vi "test BC to RT with Start Stop and Status.vi"(8 "error in":errorcluster, 11 "Loopback in":refnum<class "Loopback.lvclass">) -> (0 "error out":errorcluster, 3 "Loopback out":refnum<class "Loopback.lvclass">)   [LabVIEW 2020, in "Loopback.lvclass"]
uses:
  Loopback.lvclass
  C:/Users/nitest/Desktop/Git 2020/niveristand-custom-device-testing-tools/VeriStandTestCase/VeriStandTestCase.lvclass
  <vilib>/numeric/Random Number (Range) U64.vi
  8be00f4c-25bf-4da0-90d8-0b538b3cd633.vi
  2563bb73-47aa-45b7-be38-1c5e71b75716.vi
  <vilib>/numeric/sub_Random U32.vi
  <vilib>/NI VeriStand/Execution/Workspace/NI VeriStand - Set Single Channel Value.vi
  <vilib>/NI VeriStand/Execution/Workspace/NI VeriStand - Set Multiple Channel Values.vi
  <vilib>/NI VeriStand/Execution/Workspace/NI VeriStand - Get Multiple Channel Values.vi
  niveristand-custom-device-testing-tools/VeriStandTestUtilities/VeriStandTestUtilities.lvlib
  <vilib>/NI VeriStand/Execution/Workspace/NI_VS Workspace ExecutionAPI.lvlib
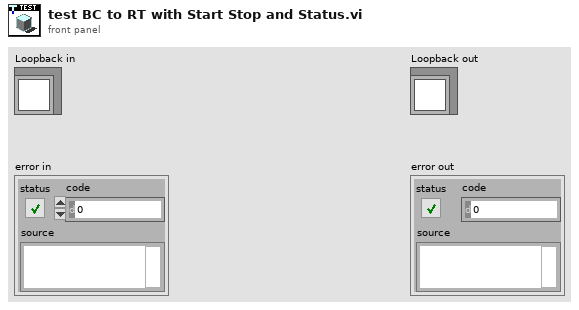
[diagram p1: front panel]
types:
  T1 = typedef "NI_VS Workspace ExecutionAPI.lvlib/WorkspaceAPI.ctl" = refnum<k24>
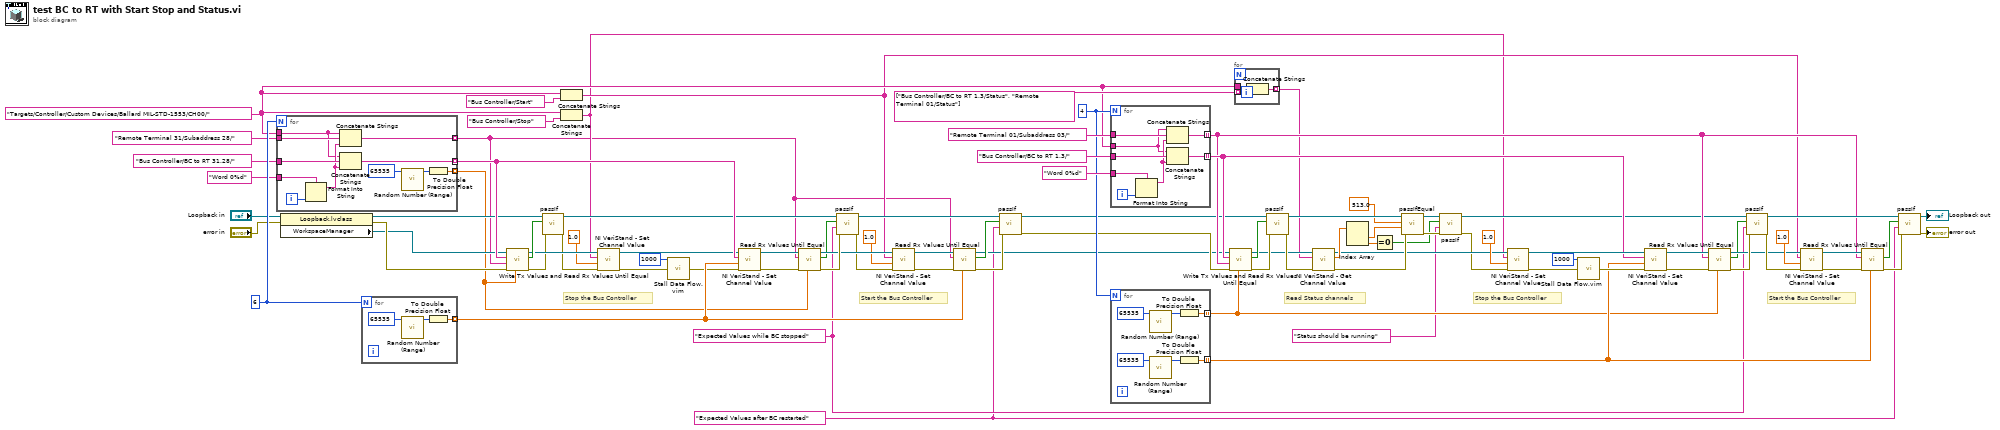
[diagram p0: block diagram]
diagram:
  w13 = "Targets/Controller/Custom Devices/Ballard MIL-STD-1553/CH00/" ("base name for channel aliases")
  w1 = "Expected Values after BC restarted" ("Channel")
  w2 = "Expected Values while BC stopped" ("Channel")
  w45 = 4
  w77 = 6
  # "Read Status channels"
  # "Start the Bus Controller"
  # "Stop the Bus Controller"
  # "Start the Bus Controller"
  # "Stop the Bus Controller"
  n1 = for {
    N: w77 -> [_]
    tunnel: "Bus Controller/BC to RT 31.28/" ("Channel") -> [w101]
    tunnel: [w102] -> w78 mode=indexing
    tunnel: "Remote Terminal 31/Subaddress 28/" ("Channel") -> [w100]
    tunnel: [w99] -> w5 mode=indexing
    tunnel: "Word 0%d" -> [w97]
    tunnel: [w93] -> w57 mode=indexing
    tunnel: w13 -> [w92]
    i -> [w98]
    n2 = Format Into String(format string=w97, w98) -> (resulting string=w96:string)  [unwired: 2 in, 1 out]
    n3 = Concatenate Strings(w92, w100, w96) -> (w99:string)
    n4 = Concatenate Strings(w92, w101, w96) -> (w102:string)
    n5 = call-poly <vilib>:"Random Number (Range).vi"("upper bound (100)"=u64 65535) -> ("number"=w95:u64)  [unwired: 10 in]
    n6 = To Double Precision Float(number=w95) -> (double precision float=w93:dbl)
  }
  n7 = property class="Loopback.lvclass"(reference="Loopback in", error in="error in") -> (reference out=w59:refnum<class "Loopback.lvclass">, error out=w60:errorcluster, "WorkspaceManager"=w58:T1)
  n8 = for {
    N: w77 -> [_]
    tunnel: [w103] -> w89 mode=indexing
    n9 = call-poly <vilib>:"Random Number (Range).vi"("upper bound (100)"=u64 65535) -> ("number"=w104:u64)  [unwired: 10 in]
    n10 = To Double Precision Float(number=w104) -> (double precision float=w103:dbl)
  }
  n11 = call "Write Tx Values and Read Rx Values Until Equal.vi"("Tx values"=w57, "error in"=w60, "Rx aliases"=w5, "Tx aliases"=w78, "workspace manager in"=w58) -> ("error out"=w79:errorcluster, "values equal"=w81:bool, "workspace manager out"=w80:T1)  [unwired: 4 in]
  n12 = call-dynamic "passIf.vi"("error in (no error)"=w79, "pass"=w81, "TestCase in"=w59) -> ("error out"=w75:errorcluster, "TestCase out"=w76:refnum<class "Loopback.lvclass">)  [unwired: 7 in]
  n13 = Concatenate Strings(w13, "Bus Controller/Start" ("Channel")) -> (w9:string)
  n14 = Concatenate Strings(w13, "Bus Controller/Stop" ("Channel")) -> (w8:string)
  n15 = call-poly <vilib>:"NI VeriStand - Set Channel Value.vi"("error in (no error)"=w75, "Value"=1.0, "Channel"=w8, "WorkspaceManager in"=w80) -> ("error out"=w67:errorcluster, "WorkspaceManager out"=w73:T1)  [unwired: 6 in]
  n16 = call "Stall Data Flow.vim"("value in"=w67, "milliseconds to wait"=u32 1000) -> ("value out"=w66:errorcluster)  [unwired: 1 out]
  n17 = call-poly <vilib>:"NI VeriStand - Set Channel Value.vi"("error in (no error)"=w66, "Values"=w89, "Channels"=w78, "WorkspaceManager in"=w73) -> ("error out"=w83:errorcluster, "WorkspaceManager out"=w82:T1)  [unwired: 6 in]
  n18 = call "Read Rx Values Until Equal.vi"("expected values"=w57, "error in"=w83, "Rx aliases"=w5, "workspace manager in"=w82) -> ("error out"=w85:errorcluster, "values equal expected"=w4:bool, "workspace manager out"=w84:T1)  [unwired: 5 in]
  n19 = call-dynamic "passIf.vi"("error in (no error)"=w85, "message (\"\")"=w2, "pass"=w4, "TestCase in"=w76) -> ("error out"=w70:errorcluster, "TestCase out"=w69:refnum<class "Loopback.lvclass">)  [unwired: 6 in]
  n20 = call-poly <vilib>:"NI VeriStand - Set Channel Value.vi"("error in (no error)"=w70, "Value"=1.0, "Channel"=w9, "WorkspaceManager in"=w84) -> ("error out"=w71:errorcluster, "WorkspaceManager out"=w86:T1)  [unwired: 6 in]
  n21 = call "Read Rx Values Until Equal.vi"("expected values"=w89, "error in"=w71, "Rx aliases"=w5, "workspace manager in"=w86) -> ("error out"=w88:errorcluster, "values equal expected"=w87:bool, "workspace manager out"=w10:T1)  [unwired: 5 in]
  n22 = call-dynamic "passIf.vi"("error in (no error)"=w88, "message (\"\")"=w1, "pass"=w87, "TestCase in"=w69) -> ("error out"=w12:errorcluster, "TestCase out"=w11:refnum<class "Loopback.lvclass">)  [unwired: 6 in]
  n23 = for {
    N: w45 -> [_]
    tunnel: "Bus Controller/BC to RT 1.3/" ("Channel") -> [w112]
    tunnel: [w113] -> w39 mode=indexing
    tunnel: "Remote Terminal 01/Subaddress 03/" ("Channel") -> [w111]
    tunnel: [w110] -> w28 mode=indexing
    tunnel: "Word 0%d" -> [w108]
    tunnel: w13 -> [w106]
    i -> [w109]
    n24 = Format Into String(format string=w108, w109) -> (resulting string=w107:string)  [unwired: 2 in, 1 out]
    n25 = Concatenate Strings(w106, w111, w107) -> (w110:string)
    n26 = Concatenate Strings(w106, w112, w107) -> (w113:string)
  }
  n27 = for {
    N: w45 -> [_]
    tunnel: [w117] -> w27 mode=indexing
    tunnel: [w114] -> w22 mode=indexing
    n28 = call-poly <vilib>:"Random Number (Range).vi"("upper bound (100)"=u64 65535) -> ("number"=w116:u64)  [unwired: 10 in]
    n29 = call-poly <vilib>:"Random Number (Range).vi"("upper bound (100)"=u64 65535) -> ("number"=w118:u64)  [unwired: 10 in]
    n30 = To Double Precision Float(number=w116) -> (double precision float=w114:dbl)
    n31 = To Double Precision Float(number=w118) -> (double precision float=w117:dbl)
  }
  n32 = call "Write Tx Values and Read Rx Values Until Equal.vi"("Tx values"=w22, "error in"=w12, "Rx aliases"=w28, "Tx aliases"=w39, "workspace manager in"=w10) -> ("error out"=w38:errorcluster, "values equal"=w37:bool, "workspace manager out"=w36:T1)  [unwired: 4 in]
  n33 = for {
    tunnel: string[] ["Bus Controller/BC to RT 1.3/Status", "Remote Terminal 01/Status"] -> [w122] mode=indexing
    tunnel: [w121] -> w23 mode=indexing
    tunnel: w13 -> [w120]
    n34 = Concatenate Strings(w120, w122) -> (w121:string)
  }
  n35 = call-dynamic "passIf.vi"("error in (no error)"=w38, "pass"=w37, "TestCase in"=w11) -> ("error out"=w43:errorcluster, "TestCase out"=w42:refnum<class "Loopback.lvclass">)  [unwired: 7 in]
  n36 = call-poly <vilib>:"NI VeriStand - Get Channel Value.vi"("error in (no error)"=w43, "Channels"=w23, "WorkspaceManager in"=w36) -> ("error out"=w44:errorcluster, "Values"=w41:dbl[], "WorkspaceManager out"=w40:T1)  [unwired: 6 in]
  n37 = Index Array(array=w41) -> (element #1=w21:dbl, element #2=w14:dbl)  [unwired: 2 in]
  n38 = Equal To 0?(x=w14) -> (x = 0?=w15:bool)
  n39 = call-dynamic "passIfEqual.vi"("error in (no error)"=w44, "y"=w21, "x"=513.0 ("element"), "TestCase in"=w42) -> ("error out"=w18:errorcluster, "TestCase out"=w19:refnum<class "Loopback.lvclass">)  [unwired: 6 in]
  n40 = call-dynamic "passIf.vi"("error in (no error)"=w18, "message (\"\")"="Status should be running" ("Channel"), "pass"=w15, "TestCase in"=w19) -> ("error out"=w17:errorcluster, "TestCase out"=w16:refnum<class "Loopback.lvclass">)  [unwired: 6 in]
  n41 = call-poly <vilib>:"NI VeriStand - Set Channel Value.vi"("error in (no error)"=w17, "Value"=1.0, "Channel"=w8, "WorkspaceManager in"=w40) -> ("error out"=w47:errorcluster, "WorkspaceManager out"=w52:T1)  [unwired: 6 in]
  n42 = call "Stall Data Flow.vim"("value in"=w47, "milliseconds to wait"=u32 1000) -> ("value out"=w46:errorcluster)  [unwired: 1 out]
  n43 = call-poly <vilib>:"NI VeriStand - Set Channel Value.vi"("error in (no error)"=w46, "Values"=w27, "Channels"=w39, "WorkspaceManager in"=w52) -> ("error out"=w34:errorcluster, "WorkspaceManager out"=w35:T1)  [unwired: 6 in]
  n44 = call "Read Rx Values Until Equal.vi"("expected values"=w22, "error in"=w34, "Rx aliases"=w28, "workspace manager in"=w35) -> ("error out"=w33:errorcluster, "values equal expected"=w31:bool, "workspace manager out"=w32:T1)  [unwired: 5 in]
  n45 = call-dynamic "passIf.vi"("error in (no error)"=w33, "message (\"\")"=w2, "pass"=w31, "TestCase in"=w16) -> ("error out"=w50:errorcluster, "TestCase out"=w49:refnum<class "Loopback.lvclass">)  [unwired: 6 in]
  n46 = call-poly <vilib>:"NI VeriStand - Set Channel Value.vi"("error in (no error)"=w50, "Value"=1.0, "Channel"=w9, "WorkspaceManager in"=w32) -> ("error out"=w29:errorcluster, "WorkspaceManager out"=w30:T1)  [unwired: 6 in]
  n47 = call "Read Rx Values Until Equal.vi"("expected values"=w27, "error in"=w29, "Rx aliases"=w28, "workspace manager in"=w30) -> ("error out"=w26:errorcluster, "values equal expected"=w25:bool)  [unwired: 5 in, 1 out]
  n48 = call-dynamic "passIf.vi"("error in (no error)"=w26, "message (\"\")"=w1, "pass"=w25, "TestCase in"=w49) -> ("error out"=→"error out":errorcluster, "TestCase out"=→"Loopback out":refnum<class "Loopback.lvclass">)  [unwired: 6 in]
